vi "Mimic 1.vi"() -> ()   [LabVIEW 2018]
panel:
  in  "stop":bool
  in  "Polling Rate (ms)":u32
  out "Pres 5 [bar]":dbl
  out "Temp 5 [c]":dbl
  out "Flow 5 [g/s]":dbl
  out "Pres 4 [bar]":dbl
  out "Temp 4 [c]":dbl
  out "Flow 4 [g/s]":dbl
  out "Pres 3 [bar]":dbl
  out "Temp 3 [c]":dbl
  out "Flow 3 [g/s]":dbl
  out "Pres 2 [bar]":dbl
  out "Temp 2 [c]":dbl
  out "Flow 2 [g/s]":dbl
  out "Pres 1 [bar]":dbl
  out "Temp 1 [c]":dbl
  out "Flow 1 [g/s]":dbl
  # "Line 4"
  # "Line 1"
  # "Line 2"
  # "Line 3"
  # "Line 5"
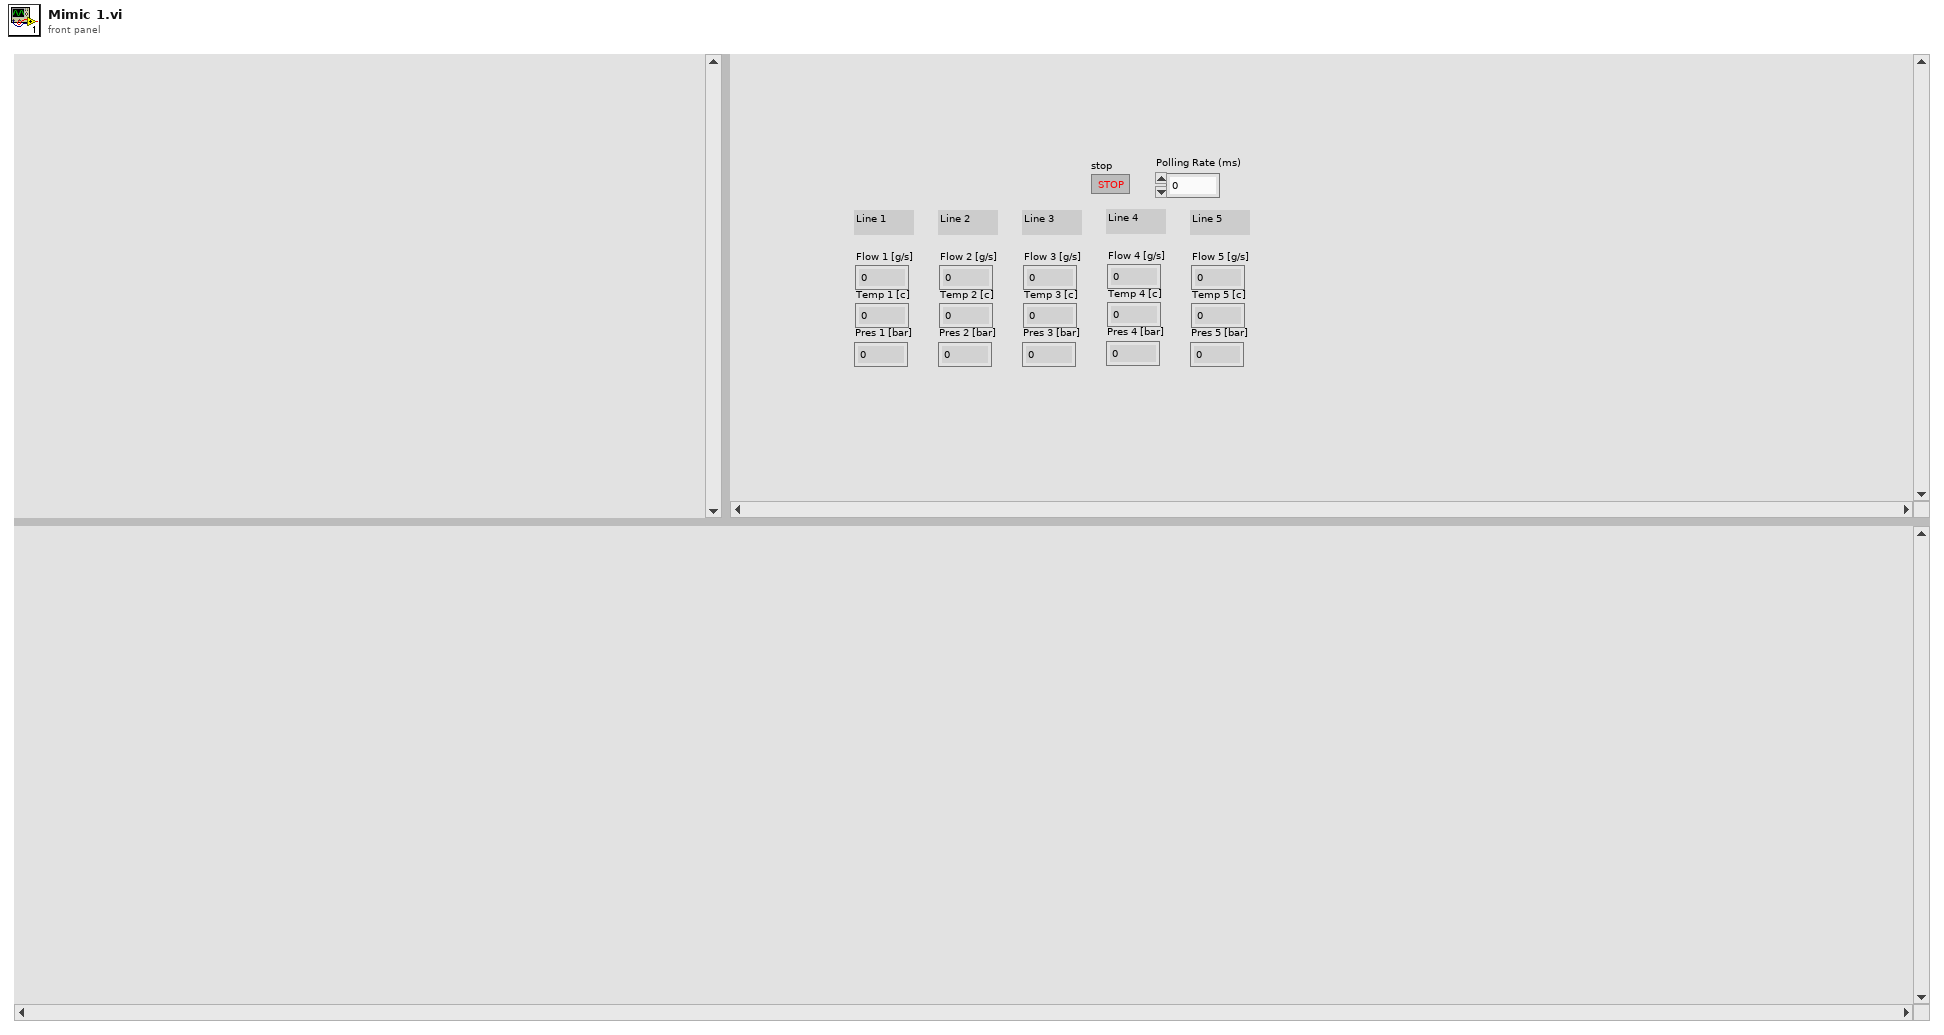
[diagram p1: front panel]
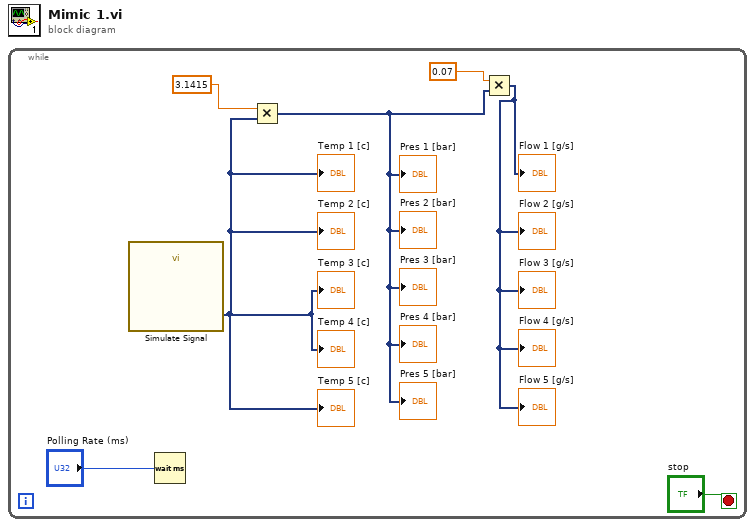
[diagram p0: block diagram]
diagram:
  n1 = while {
    stop <- "stop" stop-if-true
    n2 = call "Simulate Signal"() -> ("DC with Periodic Noise"=w4:dynamicdata)  [unwired: 14 in, 1 out]
    "Temp 1 [c]" <- w4
    "Temp 2 [c]" <- w4
    "Temp 3 [c]" <- w4
    "Temp 4 [c]" <- w4
    "Temp 5 [c]" <- w4
    n3 = Wait (ms)(milliseconds to wait="Polling Rate (ms)") -> ()  [unwired: 1 out]
    n4 = Multiply(x=3.1415 ("x*y"), y=w4) -> (x*y=w2:dynamicdata)
    "Pres 1 [bar]" <- w2
    "Pres 2 [bar]" <- w2
    "Pres 3 [bar]" <- w2
    "Pres 4 [bar]" <- w2
    "Pres 5 [bar]" <- w2
    n5 = Multiply(x=0.07 ("x*y"), y=w2) -> (x*y=→"Flow 1 [g/s]" →"Flow 2 [g/s]" →"Flow 3 [g/s]" →"Flow 4 [g/s]" →"Flow 5 [g/s]":dynamicdata)
  }
